vi "MSEncoder SubVI ApprxmSecularFreq.vi"(8 "MainRF":dbl, 9 "a":dbl, 10 "q":dbl) -> (0 "AuxRF":dbl)   [LabVIEW 2016]
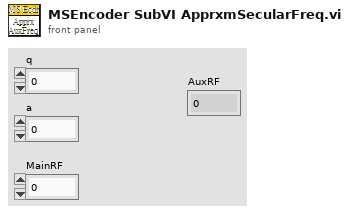
[diagram p1: front panel]
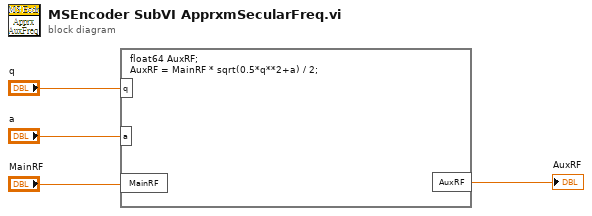
[diagram p0: block diagram]
diagram:
  n1 = formula code="float64 AuxRF;\nAuxRF = MainRF * sqrt(0.5*q**2+a) / 2;"("q"="q", "a"="a", "MainRF"="MainRF") -> ("AuxRF"=→"AuxRF":dbl)
